vi "Excel - Read Sheet.vi"(6 "Sheet(First)":i32=1, 8 "error in (no error)":errorcluster, 11 "path":path) -> (0 "error out":errorcluster, 3 "data":string[][](array[string]))   [LabVIEW 2017]
doc: "Reads a whole Excel worksheet into a two-dimensional string array. Sheet(First) selects the worksheet by index, and the application, workbook and worksheet references are opened and closed around the read."
uses:
  excel_configuration.lvlib
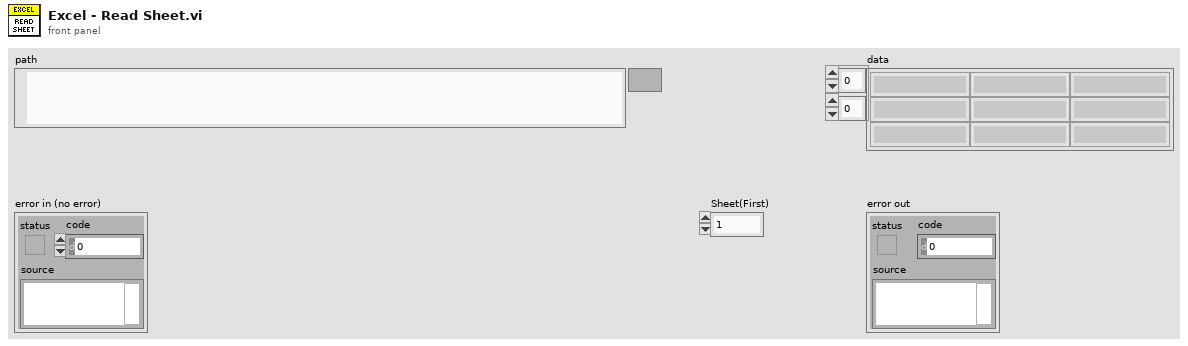
[diagram p1: front panel]
types:
  T1 = cluster{"Excel._Application":refnum<k7>, "Workbooks":refnum<k7>}
  T2 = cluster{"Excel._Application":refnum<k7>, "Workbooks":refnum<k7>, "Open":refnum<k7>}
  T3 = cluster{"Excel._Application":refnum<k7>, "Workbooks":refnum<k7>, "Open":refnum<k7>, "Worksheets":refnum<k7>, "Excel._Worksheet":refnum<k7>}
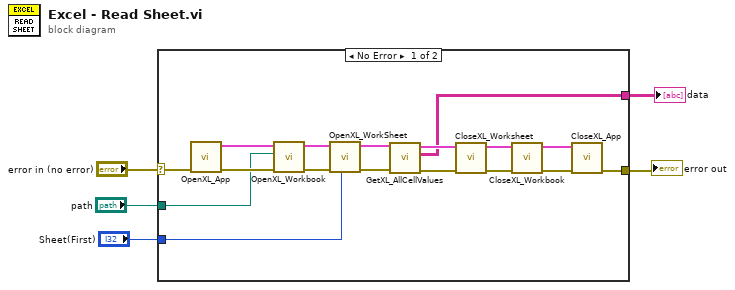
[diagram p0: block diagram]
diagram:
  n1 = case shown="No Error" "error in (no error)" {
    selector: "error in (no error)" -> [w7 w23]
    tunnel: "Sheet(First)" -> [w18 _]
    tunnel: "path" -> [w15 _]
    tunnel: [w10 w23] -> w3
    tunnel: [w6 _] -> w1
    frame No Error {
      n2 = call "OpenXL_App.vi"("error in (no error)"=w7) -> ("error out"=w16:errorcluster, "Refnum Cluster"=w17:T1)  [unwired: 9 in]
      n3 = call "OpenXL_Workbook.vi"("error in"=w16, "path"=w15, "Refnum Cluster In"=w17) -> ("error out"=w8:errorcluster, "Refnum Cluster Out"=w9:T2)  [unwired: 7 in]
      n4 = call "OpenXL_WorkSheet.vi"("Sheet"=w18, "error in (no error)"=w8, "Refnum Cluster In"=w9) -> ("error out"=w21:errorcluster, "Refnum Cluster Out"=w22:T3)  [unwired: 7 in]
      n5 = call "GetXL_AllCellValues.vi"("error in (no error)"=w21, "Refnum Cluster Out in"=w22) -> ("error out"=w13:errorcluster, "data"=w6:string[][], "Refnum Cluster Out out"=w14:T3)  [unwired: 7 in]
      n6 = call "CloseXL_Worksheet.vi"("error in (no error)"=w13, "Refnum Cluster In"=w14) -> ("error out"=w11:errorcluster, "Refnum Cluster Out"=w12:T2)  [unwired: 8 in]
      n7 = call "CloseXL_Workbook.vi"("error in (no error)"=w11, "Refnum Cluster In"=w12) -> ("error out"=w19:errorcluster, "Refnum Cluster Out"=w20:T1)  [unwired: 8 in]
      n8 = call "CloseXL_App.vi"("error in (no error)"=w19, "Refnum Cluster In"=w20) -> ("error out"=w10:errorcluster)  [unwired: 9 in]
    }
    frame Error {
    }
  }
  "error out" <- w3
  "data" <- w1
